vi "Change TTL - Ronen.vi"(6 "Pulse Duration (ms)":u32, 8 "error in (no error)":errorcluster, 9 "TTL.lvclass":refnum<class "TTL.lvclass">) -> (0 "error out":errorcluster, 1 "TTL.lvclass":refnum<class "TTL.lvclass">)   [LabVIEW 2014, in "TTL.lvclass"]
uses:
  TTL.lvclass
  TTL.lvclass/TTL.ctl
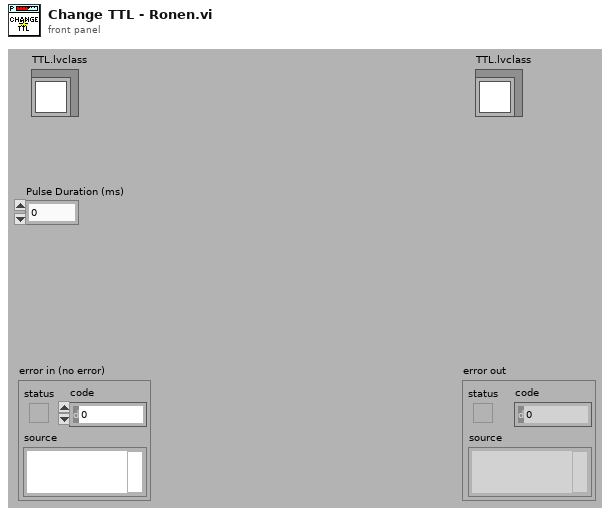
[diagram p1: front panel]
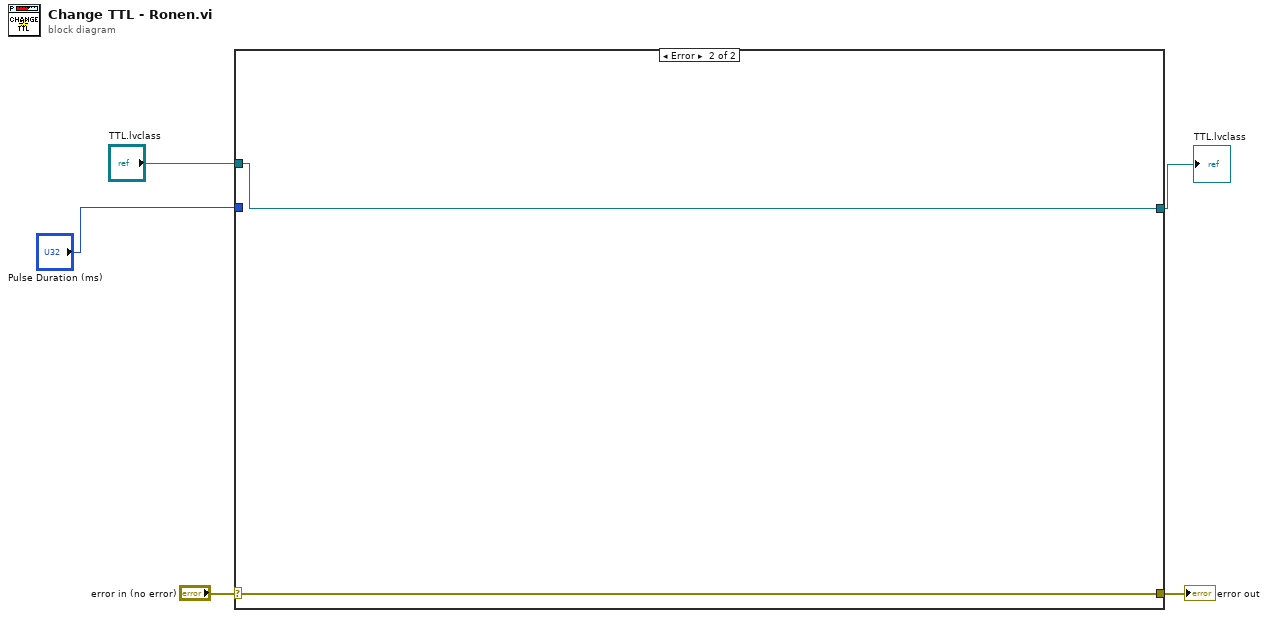
[diagram p0: block diagram]
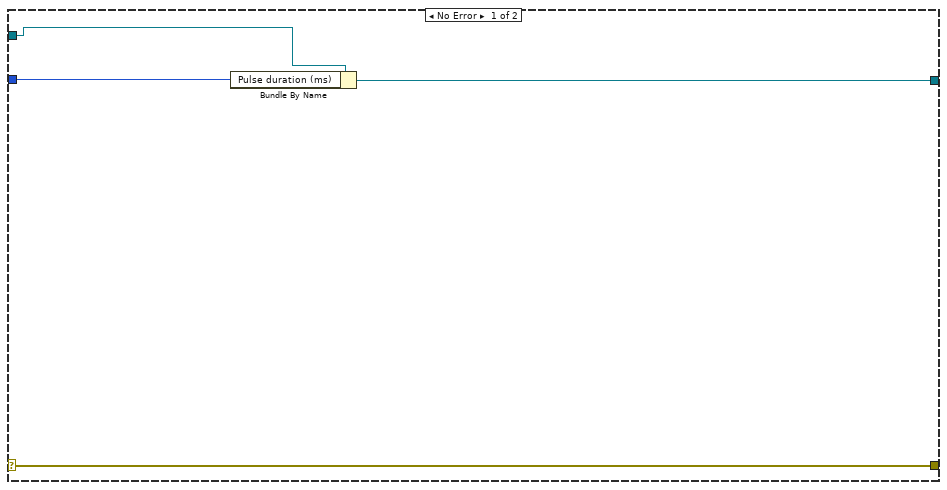
[diagram p2: hidden frame]
diagram:
  n1 = case shown="Error" "error in (no error)" {
    selector: "error in (no error)" -> [w9 w11]
    tunnel: [w9 w11] -> w4
    tunnel: "TTL.lvclass" -> [w8 w10]
    tunnel: [w7 w10] -> w2
    tunnel: "Pulse Duration (ms)" -> [w6 _]
    frame No Error {
      n2 = Bundle By Name(cluster=w8, "Pulse duration (ms)"=w6) -> (w7:refnum<class "TTL.lvclass">)
    }
    frame Error {
    }
  }
  "error out" <- w4
  "TTL.lvclass" <- w2
